vi "Handle Process Errors.vi"(8 "error in (no error)":errorcluster, 11 "Process In":refnum<class "Process.lvclass">) -> (0 "error out":errorcluster, 3 "Process Out":refnum<class "Process.lvclass">)   [LabVIEW 2020, in "Error Handler.lvclass"]
uses:
  Error Handler.lvclass
  Process/Process.lvclass
  Process/Process.lvclass/Process.ctl
  TypeDefs/Error Message Data.ctl
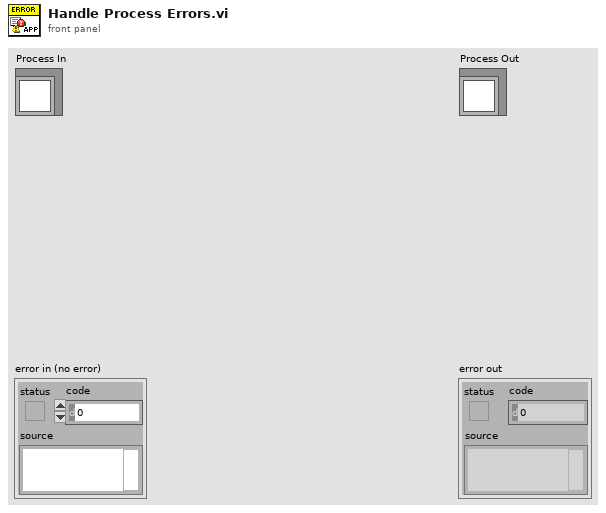
[diagram p1: front panel]
types:
  T1 = typedef "Error Handler.lvclass/Error Message Data.ctl" = cluster{"Error Type":string, "Location":string, "Error":errorcluster}
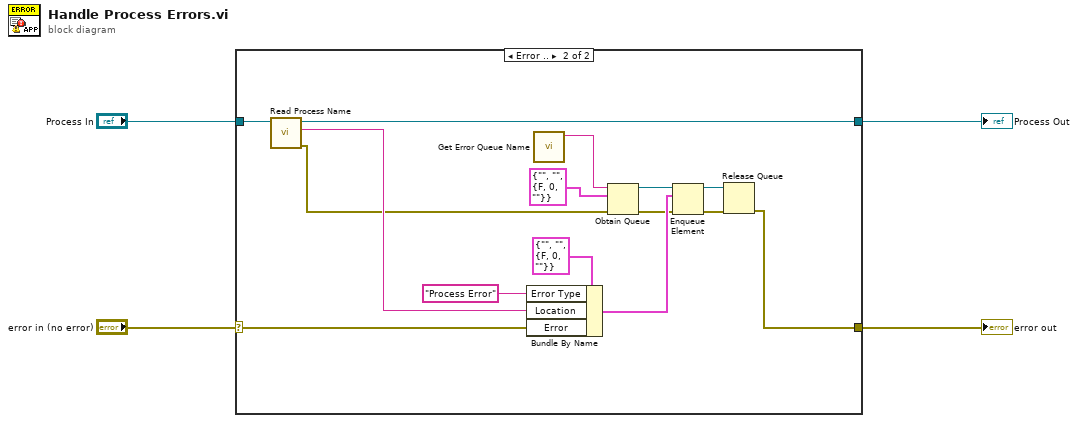
[diagram p0: block diagram]
diagram:
  n1 = case shown="Error .." "error in (no error)" {
    selector: "error in (no error)" -> [w6 w8]
    tunnel: "Process In" -> [w5 w19]
    tunnel: [w5 w20] -> w3
    tunnel: [w6 w11] -> w1
    frame No Error {
    }
    frame Error {
      n2 = call "Read Process Name.vi"("Process In"=w19) -> ("error out"=w9:errorcluster, "Process Name"=w18:string, "Process Out"=w20:refnum<class "Process.lvclass">)  [unwired: 8 in]
      n3 = Bundle By Name(cluster=T1 {"Error Type"="", "Location"="", "Error"={"status"=FALSE, "code"=0, "source"=""}} ("Error Message Data"), "Error Type"="Process Error", "Location"=w18, "Error"=w8) -> (w15:T1)
      n4 = call "Get Error Queue Name.vi"() -> ("Queue Name"=w7:string)  [unwired: 10 in, 1 out]
      n5 = Obtain Queue(name (unnamed)=w7, element data type=T1 {"Error Type"="", "Location"="", "Error"={"status"=FALSE, "code"=0, "source"=""}} ("Error Message Data"), error in (no error)=w9) -> (queue out=w16:refnum<queue>, error out=w14:errorcluster)  [unwired: 2 in, 1 out]
      n6 = Enqueue Element(queue=w16, element=w15, error in (no error)=w14) -> (queue out=w13:refnum<queue>, error out=w12:errorcluster)  [unwired: 1 in, 1 out]
      n7 = Release Queue(queue=w13, error in (no error)=w12) -> (error out=w11:errorcluster)  [unwired: 1 in, 2 out]
    }
  }
  "error out" <- w1
  "Process Out" <- w3
